vi "relative direction info.vi"(9 "central direction":dbl, 10 "direction 2":dbl, 11 "direction 1":dbl) -> (2 "direction 2 info":T1, 3 "direction 1 info":T1)   [LabVIEW 2009]
uses:
  direction info.ctl
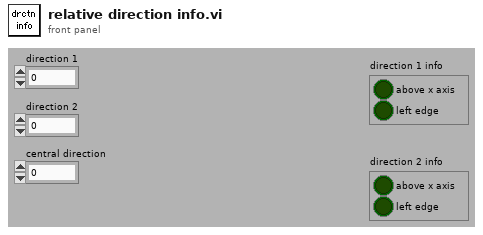
[diagram p1: front panel]
types:
  T1 = typedef "direction info.ctl" = cluster{"above x axis":bool, "left edge":bool}
  T2 = cluster{"direction 1":dbl, "direction 2":dbl, "central direction":dbl}
  T3 = cluster{"direction 1":i8, "direction 2":i8, "central direction":i8}
  T4 = cluster{"direction 1":bool, "direction 2":bool, "central direction":bool}
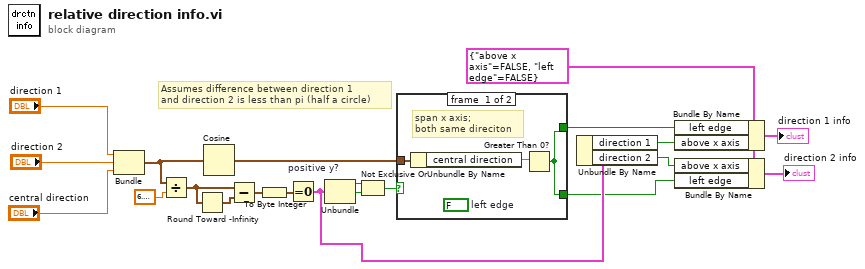
[diagram p0: block diagram]
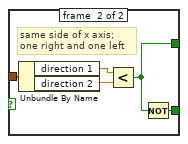
[diagram p2: hidden frame]
diagram:
  w3 = T1 {"above x axis"=FALSE, "left edge"=FALSE} ("direction 1 info")
  # "Assumes difference between direction 1\nand direction 2 is less than pi (half a circle)"
  n1 = Bundle("direction 1"="direction 1", "direction 2"="direction 2", "central direction"="central direction") -> (w11:T2)  [unwired: 1 in]
  n2 = Divide(x=w11, y=6.283185307179586) -> (x/y=w16:T2)
  n3 = Round Toward -Infinity(1:w16) -> (0:w21:T2)
  n4 = Cosine(x=w11) -> (cos(x)=w9:T2)
  n5 = Subtract(x=w16, y=w21) -> (x-y=w14:T2)
  n6 = To Byte Integer(number=w14) -> (8bit integer=w15:T3)
  n7 = Equal To 0? "positive y?"(x=w15) -> (x = 0?=w6:T4)
  n8 = Unbundle(w6) -> ("direction 1"=w13:bool, "direction 2"=w12:bool)  [unwired: 1 out]
  n9 = Not Exclusive Or(1:w12, 2:w13) -> (0:w10:bool)
  n10 = case shown="True" w10 {
    tunnel: w9 -> [w24 w29]
    tunnel: [w22 w26] -> w8
    tunnel: [w22 w25] -> w5
    frame #0 {
      (unwired) FALSE  # left edge
      # "span x axis;\nboth same direciton"
      n11 = Unbundle By Name(w24) -> ("central direction"=w23:dbl)
      n12 = Greater Than 0?(x=w23) -> (x > 0?=w22:bool)
    }
    frame #1 {
      # "same side of x axis;\none right and one left"
      n13 = Unbundle By Name(w29) -> ("direction 1"=w28:dbl, "direction 2"=w27:dbl)
      n14 = Less?(x=w28, y=w27) -> (x < y?=w26:bool)
      n15 = Not(x=w26) -> (.not. x?=w25:bool)
    }
  }
  n16 = Unbundle By Name(w6) -> ("direction 1"=w4:bool, "direction 2"=w2:bool)
  n17 = Bundle By Name(cluster=w3, "left edge"=w8, "above x axis"=w4) -> (→"direction 1 info":T1)
  n18 = Bundle By Name(cluster=w3, "above x axis"=w2, "left edge"=w5) -> (→"direction 2 info":T1)
